vi "存储.vi"   [LabVIEW 2018]
types:
  T1 = enum16{"open", "replace", "create", "open or create", "replace or create", "replace or create with confirmation"}
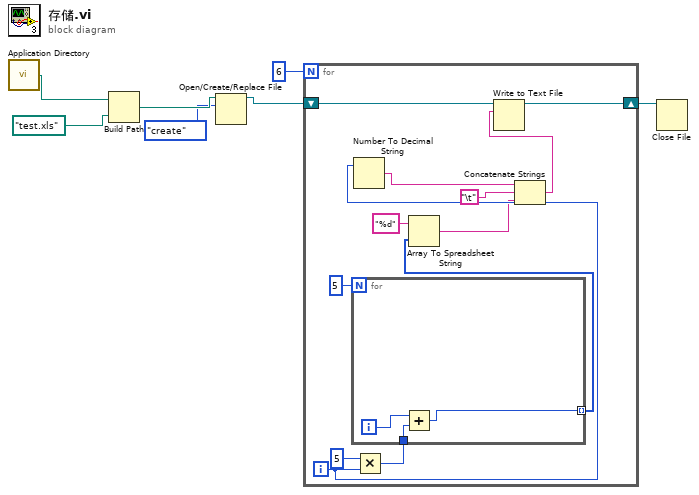
[diagram p0: block diagram]
diagram:
  n1 = call <vilib>:"Application Directory.vi"() -> ("Application Directory"=w7:path)
  n2 = Build Path(base path=w7, name or relative path=path "test.xls") -> (appended path=w5:path)
  n3 = Open/Create/Replace File(file path (use dialog)=w5, operation (0:open)=T1."create" ("操作(0:open)")) -> (refnum out=w2:refnum<file>)  [unwired: 4 in, 2 out]
  n4 = for {
    N: 6 -> [_]
    shift-right: [w13] -> w1
    shift-left: w2 -> [w14]
    i -> [w12]
    n5 = Number To Decimal String(number=w12) -> (decimal integer string=w11:string)  [unwired: 1 in]
    n6 = Multiply(x=5, y=w12) -> (x*y=w17:i32)
    n7 = for {
      N: 5 -> [_]
      tunnel: w17 -> [w22]
      tunnel: [w20] -> w16 mode=indexing
      i -> [w21]
      n8 = Add(x=w21, y=w22) -> (x+y=w20:i32)
    }
    n9 = Array To Spreadsheet String(array=w16, 3:"%d" ("格式字符串")) -> (spreadsheet string=w9:string)  [unwired: 1 in]
    n10 = Concatenate Strings(w11, "\t", w9) -> (w8:string)
    n11 = Write to Text File(file (use dialog)=w14, text=w8) -> (refnum out=w13:refnum<file>)  [unwired: 2 in, 2 out]
  }
  n12 = Close File(refnum=w1) -> ()  [unwired: 1 in, 2 out]
